vi "Initialize.vi"(7 "Process ID":string, 8 "error in (no error)":errorcluster, 11 "TCP Process in":refnum<class "TCP Process.lvclass">) -> (0 "error out":errorcluster, 3 "TCP Process out":refnum<class "TCP Process.lvclass">)   [LabVIEW 2019, in "TimingDRV Engine.lvlib" / "TCP Process.lvclass"]
uses:
  TCP Process.lvclass
  C:/Users/nitest/Desktop/CD Project Tools/Source/Engine/Parent Classes/Process/Process.lvclass
  Parent Classes/Process/Process.lvclass/Process.ctl
  TCP Process.lvclass/TCP Process.ctl
  Parent Classes/Process/Process.lvclass
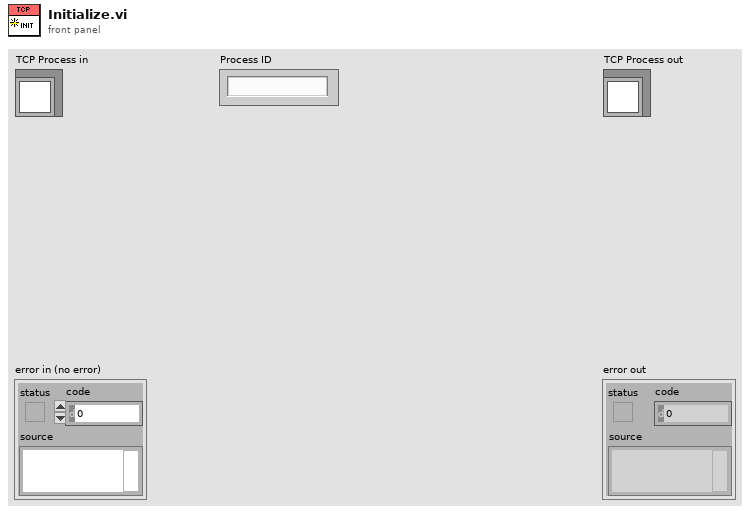
[diagram p1: front panel]
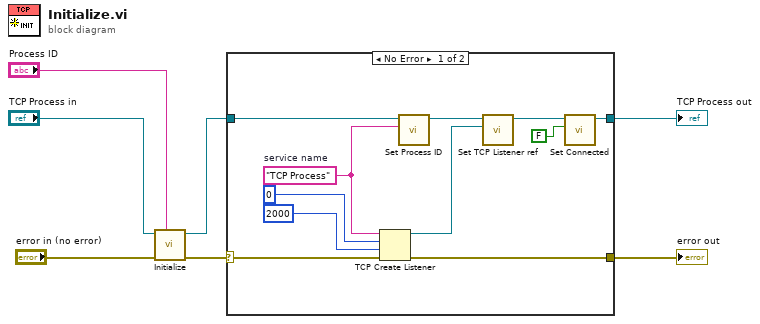
[diagram p0: block diagram]
diagram:
  n1 = call-parent "Initialize.vi"("Process ID"="Process ID", "error in (no error)"="error in (no error)", "Process in"="TCP Process in") -> ("error out"=w4:errorcluster, "Process out"=w3:refnum<class "TCP Process.lvclass">)  [unwired: 7 in]
  n2 = case shown="No Error" w4 {
    selector: w4 -> [w18 w19]
    tunnel: w3 -> [w16 w20]
    tunnel: [w12 w19] -> w1
    tunnel: [w9 w20] -> w2
    frame No Error {
      w15 = "TCP Process"  # service name
      n3 = TCP Create Listener(8:w18, 9:2000 ("timeout ms (25000)"), 10:u16 0 ("port"), 11:w15) -> (0:w12:errorcluster, 3:w13:refnum<k5>)  [unwired: 1 in, 1 out]
      n4 = call "Set Process ID.vi"("Process ID"=w15, "CD_Process in"=w16) -> ("CD_Process out"=w14:refnum<class "TCP Process.lvclass">)  [unwired: 9 in]
      n5 = call "Set TCP Listener ref.vi"("Connection ref"=w13, "TCP Process in"=w14) -> ("TCP Process out"=w10:refnum<class "TCP Process.lvclass">)  [unwired: 9 in]
      n6 = call "Set Connected.vi"("Connected"=FALSE, "TCP Process in"=w10) -> ("TCP Process out"=w9:refnum<class "TCP Process.lvclass">)  [unwired: 9 in]
    }
    frame Error {
    }
  }
  "error out" <- w1
  "TCP Process out" <- w2
